vi "Test Sinewave Class.vi"(8 "error in":errorcluster, 11 "TestCase in":refnum<class "Test FGEN.lvclass">) -> (0 "error out":errorcluster, 3 "TestCase out":refnum<class "Test FGEN.lvclass">)   [LabVIEW 2020, in "Test FGEN.lvclass"]
uses:
  Test FGEN.lvclass
  Libraries/FGen/Generador/Generador.lvclass
  <vilib>/addons/_JKI Toolkits/VI Tester/TestCase.llb/TestCase.lvclass
  <vilib>/measure/NI_MABase.lvlib
  C:/Program Files (x86)/National Instruments/LabVIEW 2020/vi.lib/addons/_JKI Toolkits/VI Tester/TestCase.llb/TestCase.lvclass
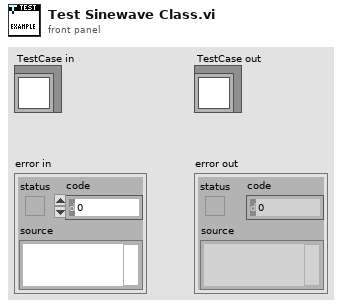
[diagram p1: front panel]
types:
  T1 = enum16{"Sine Wave", "Triangle Wave", "Square Wave", "Sawtooth Wave"}
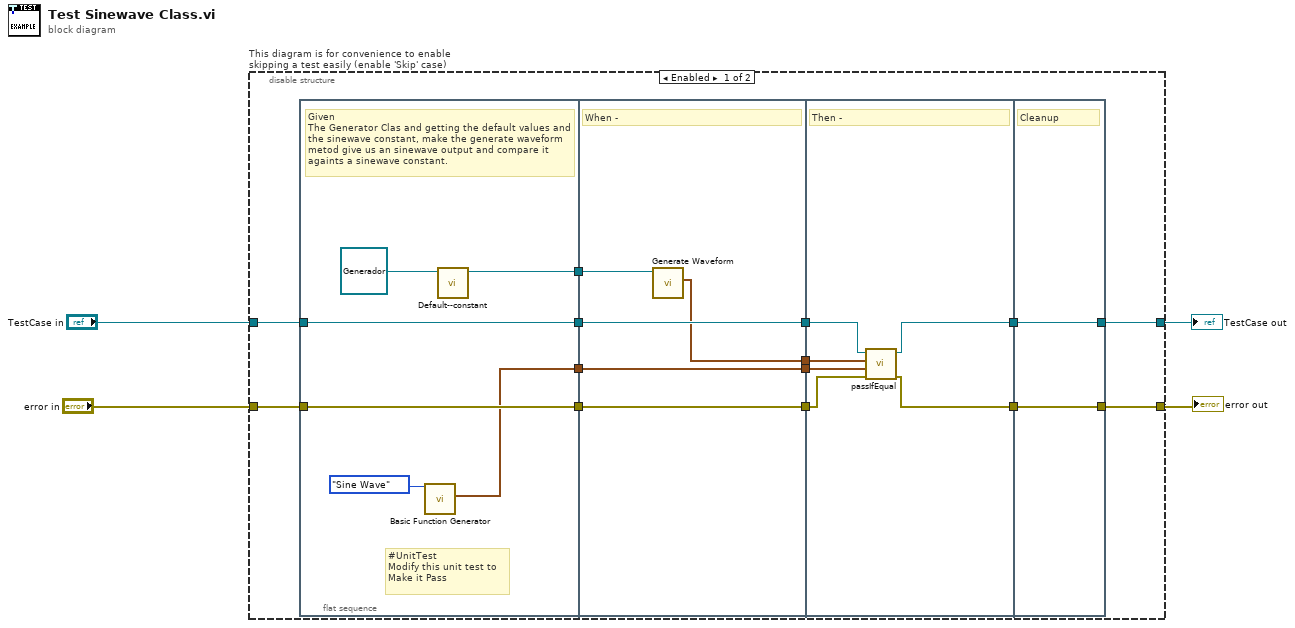
[diagram p0: block diagram]
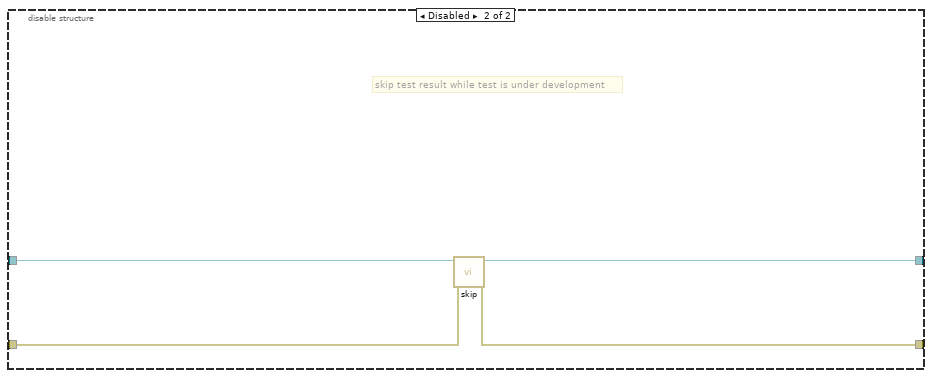
[diagram p2: hidden frame]
diagram:
  n1 = disable-structure "This diagram is for convenience to enable skipping a test easily (enable 'Skip' case)" shown="Enabled" {
    disable-tunnel: "TestCase in" -> [w10 w39]
    disable-tunnel: [w9 w38] -> w1
    disable-tunnel: [w17 w41] -> w3
    disable-tunnel: "error in" -> [w16 w40]
    frame Enabled {
      n2 = flat-sequence {
        tunnel: w10 -> [w23]
        tunnel: [w23] -> w13
        tunnel: w16 -> [w24]
        tunnel: [w24] -> w14
        tunnel: [w21] -> w8
        tunnel: [w20] -> w5
        tunnel: [w28] -> w12
        tunnel: w13 -> [w28]
        tunnel: [w29] -> w15
        tunnel: w14 -> [w29]
        tunnel: w8 -> [w27]
        tunnel: [w25] -> w7
        tunnel: [w26] -> w6
        tunnel: w5 -> [w26]
        tunnel: [w32] -> w11
        tunnel: [w35] -> w18
        tunnel: w12 -> [w33]
        tunnel: w15 -> [w34]
        tunnel: w7 -> [w31]
        tunnel: w6 -> [w30]
        tunnel: [w37] -> w17
        tunnel: [w36] -> w9
        tunnel: w11 -> [w36]
        tunnel: w18 -> [w37]
        frame #0 {
          # "#UnitTest\nModify this unit test to\nMake it Pass"
          # "Given\nThe Generator Clas and getting the default values and the sinewave constant, make the generate waveform metod give us an sinewave output and compare it againts a sinewave constant."
          n3 = call <vilib>:"Basic Function Generator.vi"("signal type"=T1."Sine Wave") -> ("signal out"=w20:waveform(dbl))  [unwired: 8 in, 2 out]
          n4 = call-dynamic "Default--constant.vi"("Generator in"=refnum<class "Generador.lvclass"> refnum ("FGen.lvlib:Generator")) -> ("Generator out"=w21:refnum<class "Generador.lvclass">)  [unwired: 9 in, 1 out]
        }
        frame #1 {
          # "When -"
          n5 = call "Generate Waveform.vi"("Generator in"=w27) -> ("Waveform"=w25:waveform(dbl))  [unwired: 8 in, 2 out]
        }
        frame #2 {
          # "Then -"
          n6 = call-dynamic "passIfEqual.vi"("error in (no error)"=w34, "y"=w30, "x"=w31, "TestCase in"=w33) -> ("error out"=w35:errorcluster, "TestCase out"=w32:refnum<class "Test FGEN.lvclass">)  [unwired: 6 in]
        }
        frame #3 {
          # "Cleanup"
        }
      }
    }
    frame Disabled {
      # "skip test result while test is under development"
      n7 = call <vilib>:"skip.vi"("error in (no error)"=w40, "TestCase in"=w39) -> ("error out"=w41:errorcluster, "TestCase out"=w38:refnum<class "Test FGEN.lvclass">)  [unwired: 8 in]
    }
  }
  "error out" <- w3
  "TestCase out" <- w1
